vi "Self-Test.vi"(8 "error in":errorcluster, 11 "Resource":string="PXI2::15::INSTR") -> (0 "error out":errorcluster, 3 "Result":string)   [LabVIEW 2020, in "PI PXI40.lvlib"]
uses:
  PI PXI40.lvlib
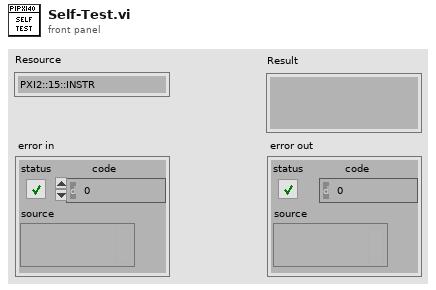
[diagram p1: front panel]
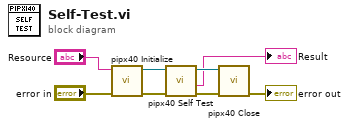
[diagram p0: block diagram]
diagram:
  n1 = call <instrlib>:"pipx40 Initialize.vi"("error in (no error)"="error in", "resource name"="Resource") -> ("error out"=w8:errorcluster, "instrument handle out"=w5:refnum<visa-resource-name>)  [unwired: 8 in]
  n2 = call <instrlib>:"pipx40 Self Test.vi"("error in (no error)"=w8, "instrument handle"=w5) -> ("error out"=w7:errorcluster, "test message"=→"Result":string, "instrument handle out"=w6:refnum<visa-resource-name>)  [unwired: 6 in, 1 out]
  n3 = call <instrlib>:"pipx40 Close.vi"("error in (no error)"=w7, "instrument handle"=w6) -> ("error out"=→"error out":errorcluster)  [unwired: 9 in]
